vi "Teleop.vi"(10 "Match Info":T1={"Autonomous Elapsed Seconds"=0.0, "TeleOp Elapsed Seconds"=0.0, "Disabled Elapsed Seconds"=0.0, "Visited Autonomous"=FALSE, "Visited TeleOp"=FALSE, "Visited Disabled"=FALSE, "Autonomous Settings"={"Autonomous Style"=enum."Independent", "VI Refnum"=refnum}}, 11 "Call Context":T2) -> ()   [LabVIEW 2012]
doc: "This VI is called for each TeleOp packet received from the DS where the robot is not disabled. It is often used to read from the joysticks and update I/O or to update setpoints for timed control loops. It should complete and return within 20 milliseconds or it may miss DS packets."
uses:
  <vilib>/Rock Robotics/WPI/DriverStation/WPI_DriverStationDerivedRobotMode.ctl
  <vilib>/Rock Robotics/WPI/DriverStation/WPI_DriverStationMatch Info.ctl
  Robot Global Data.vi
  <vilib>/Rock Robotics/Network Tables/SD Write Boolean.vi
  <vilib>/Rock Robotics/WPI/Joystick/WPI_JoystickGetSetRefNum.vi
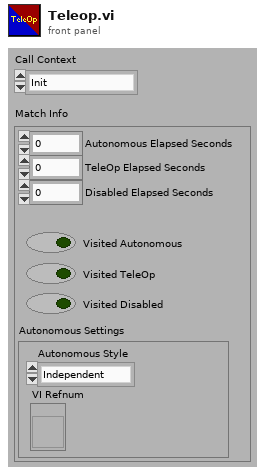
[diagram p1: front panel]
types:
  T1 = typedef "WPI_DriverStationMatch Info.ctl" = cluster{"Autonomous Elapsed Seconds":dbl, "TeleOp Elapsed Seconds":dbl, "Disabled Elapsed Seconds":dbl, "Visited Autonomous":bool, "Visited TeleOp":bool, "Visited Disabled":bool, "Autonomous Settings":cluster{"Autonomous Style":enum16{"Iterative", "Independent"}, "VI Refnum":refnum<vi>}}
  T2 = typedef "WPI_DriverStationDerivedRobotMode.ctl" = enum16{"Init", "Execute", "Stop"}
  T3 = enum16{"Off", "Close Pyramid 3pt", "Far Pyramid 3pt", "Feeder Shot", "UD Far 3pt Shot"}
  T4 = typedef "WPI_JoystickDevRef.ctl" = cluster{"Device":T5}
  T5 = typedef "WPI_JoystickDeviceEnum.ctl" = enum16{"USB 1", "USB 2", "USB 3", "USB 4", "Kinect 1", "Kinect 2"}
  T6 = typedef "WPI_JoystickButtonState.ctl" = cluster{"Button 1":bool, "Button 2":bool, "Button 3":bool, "Button 4":bool, "Button 5":bool, "Button 6":bool, "Button 7":bool, "Button 8":bool, "Button 9":bool, "Button 10":bool, "Button 11":bool, "Button 12":bool}
  T7 = cluster{"axis 1 (x)":dbl, "axis 2 (y)":dbl, "axis 3 (throttle)":dbl, "axis 4":dbl, "axis 5":dbl, "axis 6":dbl}
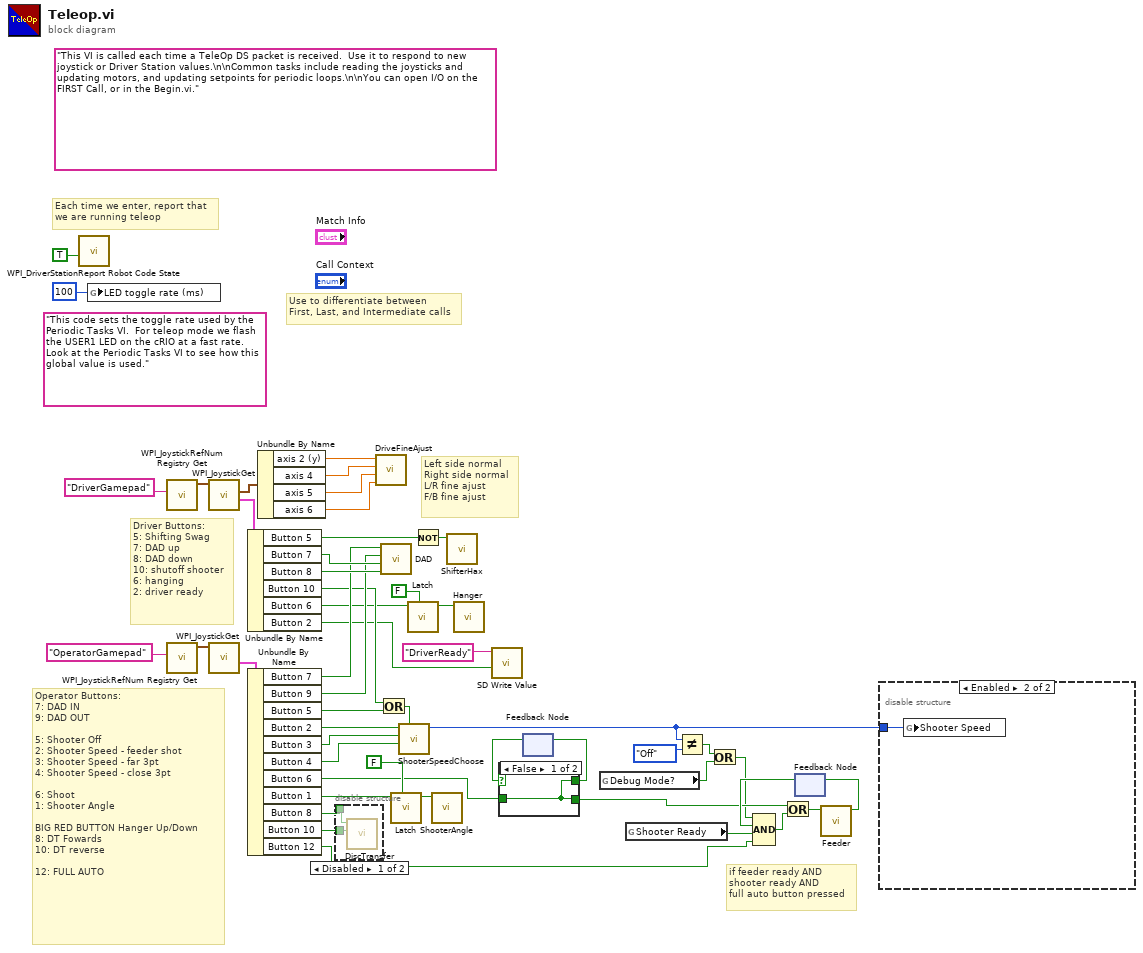
[diagram p0: block diagram]
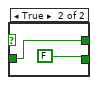
[diagram p2: hidden frame]
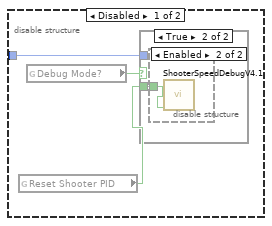
[diagram p3: hidden frame]
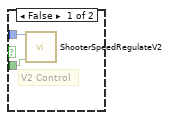
[diagram p4: hidden frame]
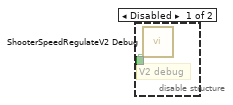
[diagram p5: hidden frame]
diagram:
  (unwired) "This code sets the toggle rate used by the Periodic Tasks VI.  For teleop mode we flash the USER1 LED on the cRIO at a fast rate.  Look at the Periodic Tasks VI to see how this global value is used."
  (unwired) "This VI is called each time a TeleOp DS packet is received.  Use it to respond to new joystick or Driver Station values.\n\nCommon tasks include reading the joysticks and updating motors, and updating setpoints for periodic loops.\n\nYou can open I/O on the FIRST Call, or in the Begin.vi."
  # "Left side normal\nRight side normal\nL/R fine ajust\nF/B fine ajust"
  # "if feeder ready AND\nshooter ready AND\nfull auto button pressed"
  # "Driver Buttons:\n5: Shifting Swag\n7: DAD up\n8: DAD down \n10: shutoff shooter\n6: hanging\n2: driver ready"
  # "Operator Buttons:\n7: DAD IN\n9: DAD OUT\n\n5: Shooter Off\n2: Shooter Speed - feeder shot\n3: Shooter Speed - far 3pt\n4: Shooter Speed - close 3pt\n\n6: Shoot\n1: Shooter Angle\n\nBIG RED BUTTON Hanger Up/Down\n8: DT Fowards\n10: DT reverse\n\n12: FULL AUTO"
  # "Each time we enter, report that\nwe are running teleop"
  # "Use to differentiate between\nFirst, Last, and Intermediate calls"
  n1 = call <vilib>:"WPI_DriverStationReport Robot Code State.vi"("TeleOp"=TRUE ("Autonomous")) -> ()  [unwired: 10 in, 1 out]
  n2 = global write "Robot Global Data.vi" "LED toggle rate (ms)"(u32 100 ("LED ms toggle rate")) -> ()
  n3 = call <vilib>:"WPI_JoystickRefNum Registry Get.vi"("refnum name"="DriverGamepad") -> ("JoystickDevRef"=w50:T4)  [unwired: 1 in, 9 out]
  n4 = call <vilib>:"WPI_JoystickRefNum Registry Get.vi"("refnum name"="OperatorGamepad") -> ("JoystickDevRef"=w45:T4)  [unwired: 1 in, 9 out]
  n5 = call <vilib>:"WPI_JoystickGet.vi"("JoystickDevRef"=w50) -> ("Buttons"=w46:T6, "Axes"=w47:T7)  [unwired: 1 in, 4 out]
  n6 = call <vilib>:"WPI_JoystickGet.vi"("JoystickDevRef"=w45) -> ("Buttons"=w44:T6)  [unwired: 1 in, 5 out]
  n7 = Unbundle By Name(w46) -> ("Button 5"=w11:bool, "Button 7"=w39:bool, "Button 8"=w38:bool, "Button 10"=w34:bool, "Button 6"=w32:bool, "Button 2"=w17:bool)
  n8 = Unbundle By Name(w44) -> ("Button 7"=w37:bool, "Button 9"=w36:bool, "Button 5"=w35:bool, "Button 2"=w29:bool, "Button 3"=w28:bool, "Button 4"=w27:bool, "Button 6"=w10:bool, "Button 1"=w33:bool, "Button 8"=w31:bool, "Button 10"=w30:bool, "Button 12"=w19:bool)
  n9 = Unbundle By Name(w47) -> ("axis 2 (y)"=w14:dbl, "axis 4"=w13:dbl, "axis 5"=w16:dbl, "axis 6"=w15:dbl)
  n10 = disable-structure shown="Disabled" {
    disable-tunnel: w31 -> [w52 _]
    disable-tunnel: w30 -> [w51 _]
    frame Disabled {
      n11 = call "DiscTransfer.vi"("DT Backwards"=w51, "DT Foward"=w52) -> ()  [unwired: 10 in]
    }
    frame Enabled {
    }
  }
  n12 = call "DriveFineAjust.vi"("Fine Ajust F/B"=w15, "Fine Ajust L/R"=w16, "Right Side Normal"=w13, "Left Side Normal"=w14) -> ()  [unwired: 8 in]
  n13 = Or(x=w34, y=w35) -> (x .or. y?=w26:bool)
  n14 = call "DAD.vi"("BAD DOWN"=w38, "BAD UP"=w39, "BAD OUT"=w36, "BAD IN"=w37) -> ()  [unwired: 7 in, 1 out]
  n15 = call "Latch.vi"("Default Value (false)"=FALSE, "Latch In"=w33) -> ("Latch Out"=w42:bool)  [unwired: 9 in]
  n16 = call "ShooterSpeedChoose.vi"("Shooter OFF"=w26, "Close 3pt Shot Button"=w27, "Far 3pt Shot Button"=w28, "Feedershot Button"=w29) -> ("Shooter Speed"=w5:T3)  [unwired: 7 in]
  n17 = call "Latch.vi"("Default Value (false)"=FALSE, "Latch In"=w32) -> ("Latch Out"=w43:bool)  [unwired: 9 in]
  n18 = Not(x=w11) -> (.not. x?=w12:bool)
  n19 = call "ShooterAngle.vi"("Shooter Angle Up?"=w42) -> ()  [unwired: 10 in, 1 out]
  n20 = call "ShifterHax.vi"("Shift low?"=w12) -> ()  [unwired: 11 in]
  n21 = call "Hanger.vi"("Hanger Up"=w43) -> ()  [unwired: 10 in, 1 out]
  n22 = call-poly <vilib>:"SD Write Value.vi"("Boolean"=w17, "Name"="DriverReady") -> ()  [unwired: 8 in, 2 out]
  n23 = feedback #1() -> (w8:bool)  [unwired: 1 in]
  n24 = case shown="False" w8 {
    tunnel: w10 -> [w53 w55]
    tunnel: [w53 w55] -> w9
    tunnel: [w53 FALSE] -> w7
    frame False {
    }
    frame True {
    }
  }
  n25 = feedback-in #1(w9) -> ()
  n26 = global read "Robot Global Data.vi" "Debug Mode?"() -> (w3:bool)
  n27 = global read "Robot Global Data.vi" "Shooter Ready"() -> (w20:bool)
  n28 = Not Equal?(x=w5, y=T3."Off" ("Shooter Speed")) -> (x != y?=w4:bool)
  n29 = Or(x=w4, y=w3) -> (x .or. y?=w2:bool)
  n30 = feedback #2() -> (w21:bool)  [unwired: 1 in]
  n31 = Compound Arithmetic op=AND(w2, w21, w20, w19) -> (w23:bool)
  n32 = Or(x=w7, y=w23) -> (x .or. y?=w24:bool)
  n33 = call "Feeder.vi"("SHOOT Button"=w24) -> ("Ready To Shoot?"=w22:bool)  [unwired: 10 in]
  n34 = feedback-in #2(w22) -> ()
  n35 = disable-structure shown="Enabled" {
    disable-tunnel: w5 -> [w58 w64]
    frame Disabled {
      n36 = global read "Robot Global Data.vi" "Reset Shooter PID"() -> (w56:bool)
      n37 = global read "Robot Global Data.vi" "Debug Mode?"() -> (w57:bool)
      n38 = case shown="True" w57 {
        tunnel: w58 -> [w60 _]
        tunnel: w56 -> [w59 w61]
        frame False {
          # "V2 Control"
          n39 = call "ShooterSpeedRegulateV2.vi"("Shooter Speed"=w60, "Reset Shooter PID"=w59) -> ()  [unwired: 12 in, 2 out]
        }
        frame True {
          n40 = disable-structure shown="Enabled" {
            disable-tunnel: w61 -> [w62 w63]
            frame Disabled {
              # "V2 debug"
              n41 = call "ShooterSpeedRegulateV2 Debug.vi"("Reset Shooter PID"=w62) -> ()  [unwired: 13 in, 2 out]
            }
            frame Enabled {
              n42 = call "ShooterSpeedDebugV4.1.vi"("Reset PID"=w63) -> ()  [unwired: 9 in, 2 out]
            }
          }
        }
      }
    }
    frame Enabled {
      n43 = global write "Robot Global Data.vi" "Shooter Speed"(w64) -> ()
    }
  }
